vi "PQfetchDataIntoFile.vi"() -> ()   [LabVIEW 2019]
uses:
  libpqlv/libpqlv.lvlib
  libpqutility.lvlib
panel:
  out "Zeitstempel":timestamp
  out "Tabellen-Bedienelement":string[][](table)
  out "DatabaseMesssageCluster":T1
  out "String":string
  in  "query":string
  out "Data":string[][](array[string])
  out "error out":errorcluster
  in  "error in":errorcluster
  out "PQnTuples":u32
  out "PQnFields":u32
  out "conn_out":u32
  out "res_out":u32
  in  "res":u32
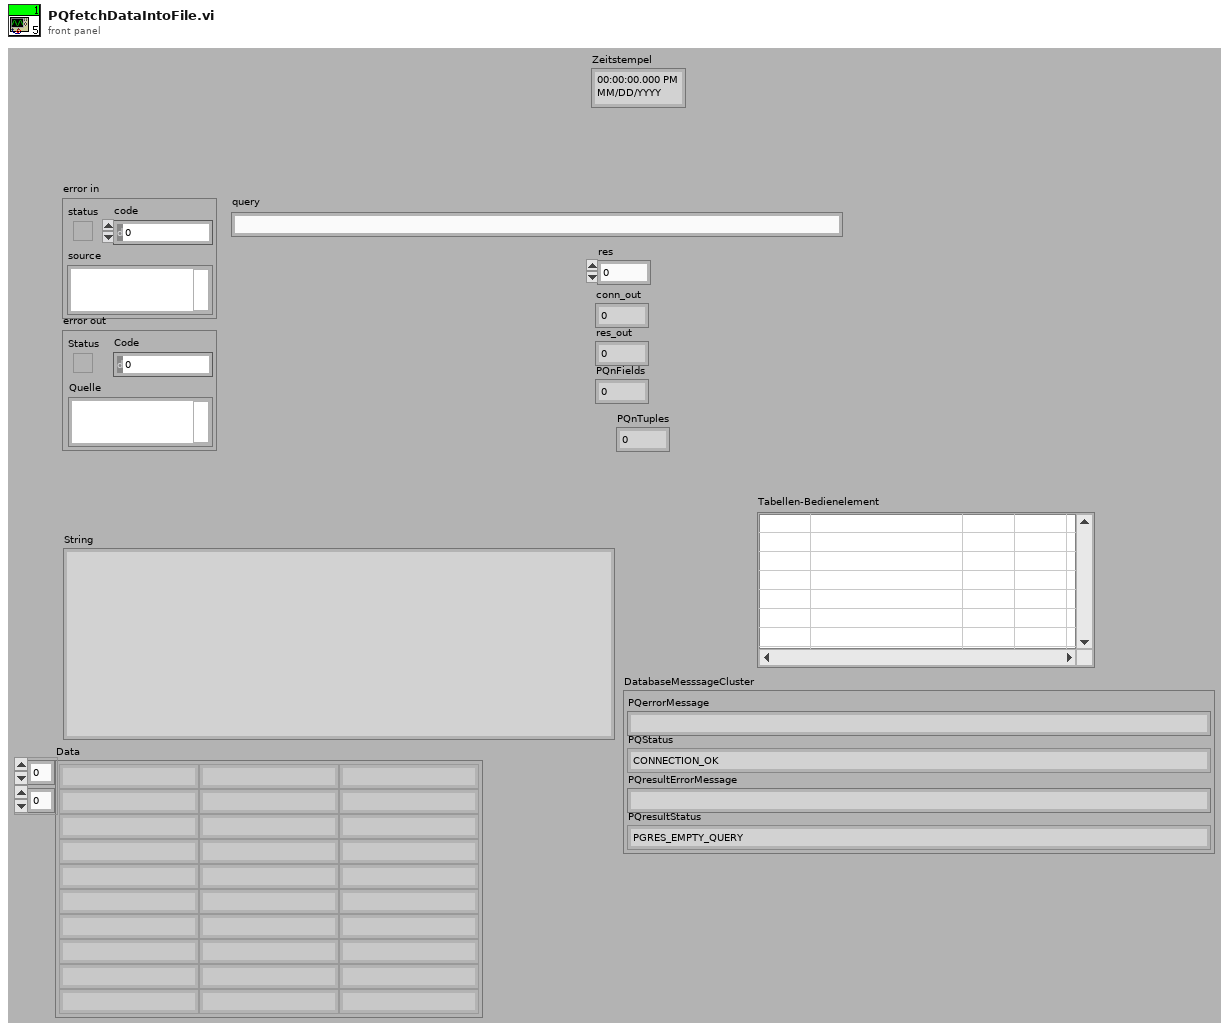
[diagram p1: front panel]
types:
  T1 = cluster{"PQerrorMessage":string, "PQStatus":enum16{"CONNECTION_OK", "CONNECTION_BAD", "CONNECTION_STARTED", "CONNECTION_MADE", "CONNECTION_AWAITING_RESPONSE", "CONNECTION_AUTH_OK", "CONNECTION_SETENV", "CONNECTION_SSL_STARTUP", "CONNECTION_NEEDED"}, "PQresultErrorMessage":string, "PQresultStatus":enum16{"PGRES_EMPTY_QUERY", "PGRES_COMMAND_OK", "PGRES_TUPLES_OK", "PGRES_COPY_OUT", "PGRES_COPY_IN", "PGRES_BAD_RESPONSE", "PGRES_NONFATAL_ERROR", "PGRES_FATAL_ERROR"}}
  T2 = enum16{"CONNECTION_OK", "CONNECTION_BAD", "CONNECTION_STARTED", "CONNECTION_MADE", "CONNECTION_AWAITING_RESPONSE", "CONNECTION_AUTH_OK", "CONNECTION_SETENV", "CONNECTION_SSL_STARTUP", "CONNECTION_NEEDED"}
  T3 = enum16{"PGRES_EMPTY_QUERY", "PGRES_COMMAND_OK", "PGRES_TUPLES_OK", "PGRES_COPY_OUT", "PGRES_COPY_IN", "PGRES_BAD_RESPONSE", "PGRES_NONFATAL_ERROR", "PGRES_FATAL_ERROR"}
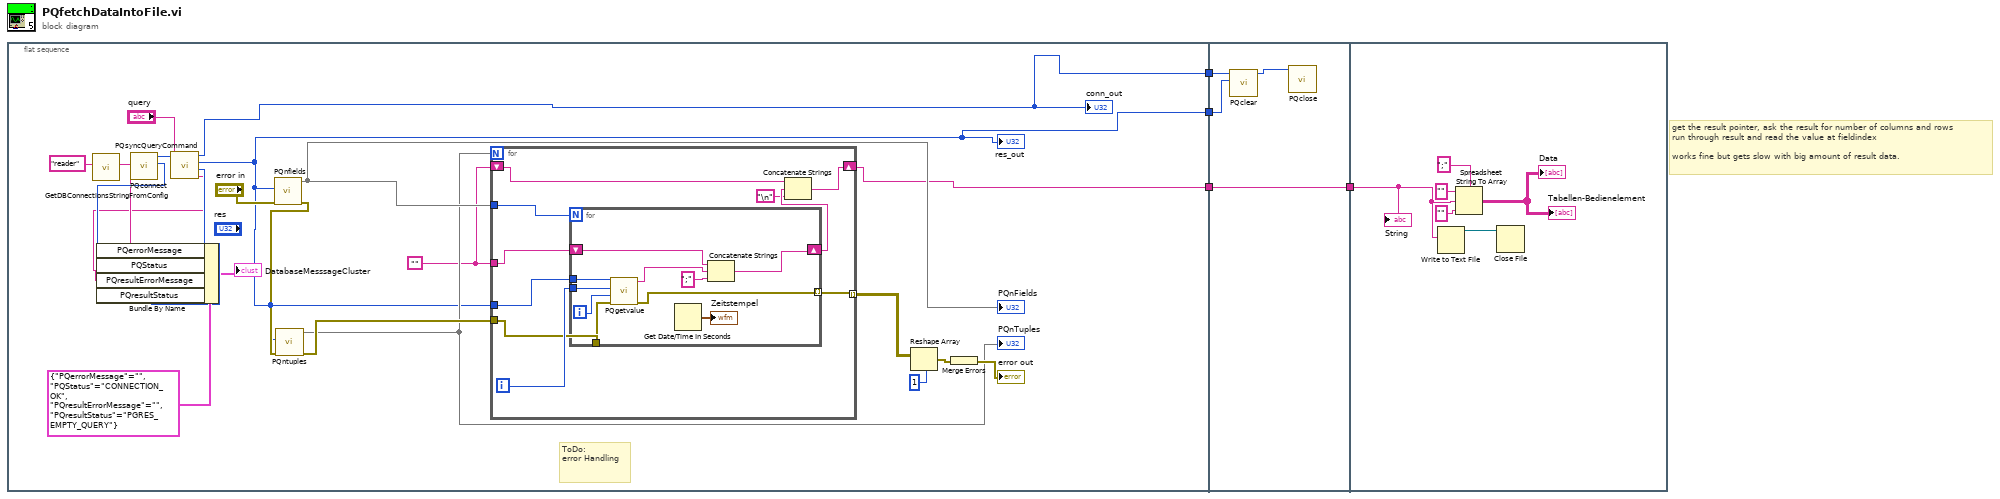
[diagram p0: block diagram]
diagram:
  # "get the result pointer, ask the result for number of columns and rows\nrun through result and read the value at fieldindex\n\nworks fine but gets slow with big amount of result data."
  n1 = flat-sequence {
    tunnel: [w14] -> w4
    tunnel: [w13] -> w3
    tunnel: [w5] -> w1
    tunnel: w4 -> [w51]
    tunnel: w3 -> [w50]
    tunnel: [w48] -> w2
    tunnel: w1 -> [w48]
    tunnel: w2 -> [w52]
    frame #0 {
      w6 = ""
      # "ToDo:\nerror Handling"
      n2 = call "GetDBConnectionsStringFromConfig.vi"("ConnectionName"="reader" ("connection_name")) -> ("DatabaseConnectionString"=w17:string)  [unwired: 10 in]
      n3 = call "PQconnect.vi"("conninfo"=w17) -> ("PQerrorMessage"=w10:string, "PQStatus"=w11:T2, "conn"=w16:u32)  [unwired: 5 in, 1 out]
      n4 = call "PQsyncQueryCommand.vi"("query"="query", "conn"=w16) -> ("PQresultErrorMessage"=w8:string, "PQresultStatus"=w9:T3, "PGresult"=w14:u32, "conn out"=w13:u32)  [unwired: 5 in]
      "res_out" <- w14
      "conn_out" <- w13
      n5 = Bundle By Name(cluster=T1 {"PQerrorMessage"="", "PQStatus"=enum."CONNECTION_OK", "PQresultErrorMessage"="", "PQresultStatus"=enum."PGRES_EMPTY_QUERY"} ("DatabaseMesssageCluster 2"), "PQerrorMessage"=w10, "PQStatus"=w11, "PQresultErrorMessage"=w8, "PQresultStatus"=w9) -> (→"DatabaseMesssageCluster":T1)
      n6 = call "PQnfields.vi"("error in (no error)"="error in", "res"=w14) -> ("error out"=w26:errorcluster, 3:w20)  [unwired: 6 in, 2 out]
      "PQnFields" <- w20
      n7 = call "PQntuples.vi"("error in (no error)"=w26, "res"=w14) -> ("error out"=w25:errorcluster, 3:w19)  [unwired: 6 in, 2 out]
      "PQnTuples" <- w19
      n8 = for {
        N: w19 -> [_]
        tunnel: w14 -> [w37]
        tunnel: w20 -> [w34]
        tunnel: w25 -> [w35]
        tunnel: [w33] -> w24 mode=indexing
        tunnel: w6 -> [w29]
        shift-right: [w31] -> w5
        shift-left: w6 -> [w30]
        i -> [w36]
        n9 = for {
          N: w34 -> [_]
          tunnel: w37 -> [w47]
          tunnel: w36 -> [w43]
          tunnel: w35 -> [w46]
          tunnel: [w45] -> w33 mode=indexing
          shift-right: [w41] -> w32
          shift-left: w29 -> [w40]
          i -> [w44]
          n10 = call "PQgetvalue.vi"("error in (no error)"=w46, "column_number"=w44, "row_number"=w43, "res"=w47) -> ("error out"=w45:errorcluster, "field_value"=w42:string)  [unwired: 6 in]
          n11 = Get Date/Time In Seconds() -> (seconds since 1Jan1904=→"Zeitstempel":timestamp)
          n12 = Concatenate Strings(w40, w42, ";" ("String")) -> (w41:string)
        }
        n13 = Concatenate Strings(w30, w32, "\n") -> (w31:string)
      }
      n14 = Reshape Array(w24, 1 ("Dimensionsgröße")) -> (w22:errorcluster[])
      n15 = Merge Errors(w22) -> (→"error out":errorcluster)
    }
    frame #1 {
      n16 = call "PQclear.vi"("res"=w51, "conn"=w50) -> ("conn_out"=w49:u32)  [unwired: 8 in, 1 out]
      n17 = call "PQclose.vi"("conn"=w49) -> ()  [unwired: 10 in, 1 out]
    }
    frame #2 {
      n18 = Write to Text File(text=w52) -> (refnum out=w53:refnum<file>)  [unwired: 3 in, 2 out]
      n19 = Spreadsheet String To Array(delimiter (Tab)=";" ("Trennzeichen (Tabulator)"), format string="" ("Format-String"), spreadsheet string=w52, array type (2D Dbl)="" ("Trennzeichen (Tabulator)")) -> (array=→"Data" →"Tabellen-Bedienelement":string[][])
      n20 = Close File(refnum=w53) -> ()  [unwired: 1 in, 2 out]
      "String" <- w52
    }
  }
